vi "Get Data DVR.vi"(8 "error in (no error)":errorcluster, 11 "Dictionary in":refnum<class "Dictionary.lvclass">) -> (0 "error out":errorcluster, 2 "Data DVR":refnum<data-value>, 3 "Dictionary out":refnum<class "Dictionary.lvclass">)   [LabVIEW 2018, in "Application.lvlib" / "Dictionary.lvclass"]
uses:
  Dictionary.lvclass
  Dictionary.lvclass/Dictionary.ctl
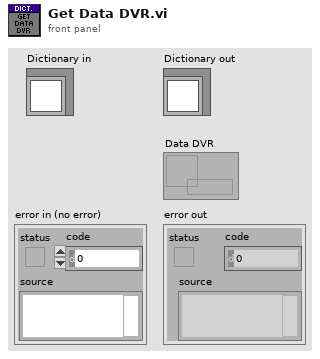
[diagram p1: front panel]
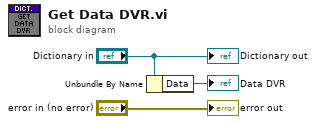
[diagram p0: block diagram]
diagram:
  n1 = Unbundle By Name("Dictionary in") -> ("Data"=→"Data DVR":refnum<data-value>)
  "error out" <- "error in (no error)"
  "Dictionary out" <- "Dictionary in"
